vi "PCO_GetFPSExposureMode.vi"(8 "error in (no error)":errorcluster {"code" format="%x"}, 11 "ph":u64) -> (0 "error out":errorcluster {"code" format="%x"}, 1 "wFPSExposureMode":u16(ring) items=["OFF", "ON"], 2 "ErrorMessage":i32 format="%x", 3 "ph out":u64, 5 "dwFPSExposureTime":u32)   [LabVIEW 2020, in "SDK.lvlib" / "TimingControl.lvlib"]
doc: "<b>Description:</b>\nThis function returns the status of FPS exposure mode setting and according exposure time information.\n\n<b>Supported camera type:</b>\npco.1200\n\n<b>Descriptor dependency:</b>\nNone"
uses:
  TimingControl.lvlib
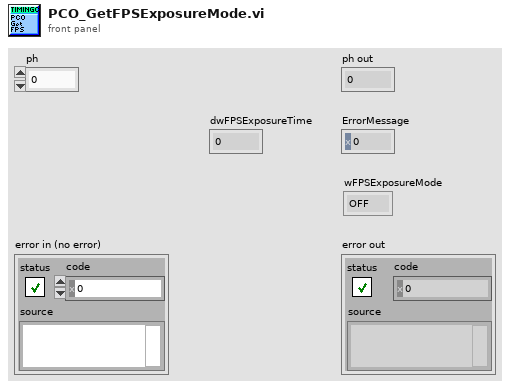
[diagram p1: front panel]
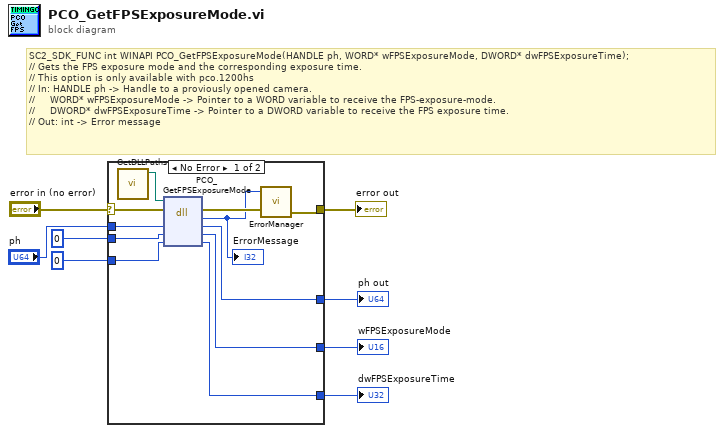
[diagram p0: block diagram]
diagram:
  # "SC2_SDK_FUNC int WINAPI PCO_GetFPSExposureMode(HANDLE ph, WORD* wFPSExposureMode, DWORD* dwFPSExposureTime);\n// Gets the FPS exposure mode and the corresponding exposure time.\n// This option is only available with pco.1200hs\n// In: HANDLE ph -> Handle to a proviously opened camera.\n//     WORD* wFPSExposureMode -> Pointer to a WORD variable to receive the FPS-exposure-mode.\n//     DWORD* dwFPSExposureTime -> Pointer to a DWORD variable to receive the FPS exposure time.\n// Out: int -> Error message"
  n1 = case shown="No Error" "error in (no error)" {
    selector: "error in (no error)" -> [w13 w23]
    tunnel: "ph" -> [w19 w22]
    tunnel: [w18 w22] -> w7
    tunnel: u16 0 ("wFPSExposureMode") -> [w17 w21]
    tunnel: [w16 w21] -> w5
    tunnel: u32 0 ("dwFPSExposureTime") -> [w15 w20]
    tunnel: [w14 w20] -> w3
    tunnel: [w11 w23] -> w2
    frame No Error {
      n2 = call "GetDLLPaths.vi"() -> ("SC2_Cam_Path"=w9:path)  [unwired: 9 in, 2 out]
      n3 = dll-call lib="?" fn="PCO_GetFPSExposureMode"(path in=w9, error in=w13, "ph"=w19, "wFPSExposureMode"=w17, "dwFPSExposureTime"=w15) -> (error out=w12:errorcluster, "return type"=w10:i32, "ph"=w18:u64, "wFPSExposureMode"=w16:u16, "dwFPSExposureTime"=w14:u32)  [unwired: 1 in, 1 out]
      "ErrorMessage" <- w10
      n4 = call "ErrorManager.vi"("error in (no error)"=w12, "error code"=w10) -> ("error out"=w11:errorcluster)  [unwired: 3 in]
    }
    frame Error {
    }
  }
  "ph out" <- w7
  "wFPSExposureMode" <- w5
  "dwFPSExposureTime" <- w3
  "error out" <- w2
